vi "3.1.1.1-VectorNav Write.vi"(10 "Command":string="$VNRRG,08*7B") -> ()   [LabVIEW 2010]
uses:
  <vilib>/rvi/interface/nirviMethod/nirviMethod.xnode
  <vilib>/userDefined/High Color/nirio_resource_hc.ctl
  <vilib>/rvi/interface/nirviOpenFPGA/nirviOpenFPGA.xnode
  <vilib>/rvi/interface/nirviCloseFPGA/nirviCloseFPGA.xnode
  <vilib>/Utility/error.llb/Error Cluster From Error Code.vi
  FPGA Bitfiles/DaveBrain_FPGATarget_1.2.1.1-VectorNa_98C397BE.lvbitx
  1-Hindbrain/1.2-Where/1.2.1-VectorNav/1.2.1.1-VectorNav Read Write.vi
  NiFpgaLv.dll
  <vilib>/rvi/errors/niLvFpgaWhatHappensToTopLevelVI.ctl
  <vilib>/rvi/interface/common/niFpgaNodeNameForErrorReporting.ctl
  <vilib>/rvi/errors/niLvFpgaAdjustHostInterfaceError.vi
  <vilib>/FPGAPlugInAG/Dynamic/niLvFpga_Close_Dynamic.vi
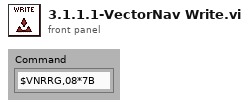
[diagram p1: front panel]
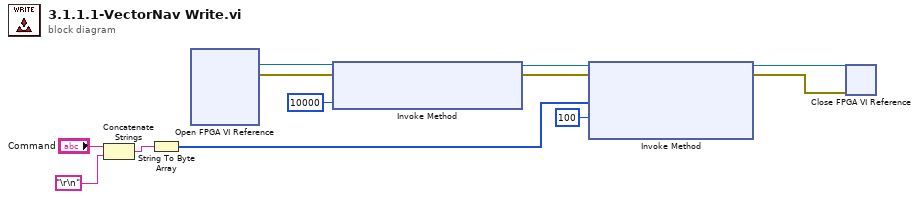
[diagram p0: block diagram]
diagram:
  n1 = Concatenate Strings("Command", "\r\n") -> (w2:string)
  n2 = String To Byte Array(string=w2) -> (unsigned byte array=w5:u8[])
  n3 = xnode "Open FPGA VI Reference"() -> ("FPGA VI Reference Out"=w11:refnum<k20>, "error out"=w12:errorcluster)  [unwired: 2 in]
  n4 = xnode "Invoke Method"("FPGA VI Reference In"=w11, "error in"=w12, "Depth"=u32 10000) -> ("FPGA VI Reference Out"=w9:refnum<k20>, "error out"=w8:errorcluster)
  n5 = xnode "Invoke Method"("FPGA VI Reference In"=w9, "error in"=w8, "Data"=w5, "Timeout (ms)"=100) -> ("FPGA VI Reference Out"=w7:refnum<k20>, "error out"=w6:errorcluster)  [unwired: 1 out]
  n6 = xnode "Close FPGA VI Reference"("FPGA VI Reference In"=w7, "error in"=w6) -> ()  [unwired: 1 out]
